vi "test_0.1.0a1.vi"() -> ()   [LabVIEW 2011]
panel:
  in  "meta":string[](array[string])
  in  "Pages":i32
  out "return type 5":i32
  out "return type 4":i32
  out "return type 3":i32
  out "return type 2":i32
  out "return type":i32
  in  "path in":path=path "\\\\vmware-host\\Shared Folders/shared/camtiff/bin/libctiff.dll"
  out "error out":errorcluster
  in  "name":string="LabVIEW"
  in  "image_desc":string="LabVIEW Testing"
  in  "software":string="Make"
  in  "model":string="Model"
  in  "make":string="Make"
  in  "copyright":string="Copyright"
  in  "artist":string="Artist"
  in  "output_file":path=path "\\\\vmware-host\\Shared Folders/shared/camtiff/labview_test.tiff"
  in  "Array":u16[][](array[numeric])=[[0, 0, 0, 0], [0, 24000, 0, 0], [0, 0, 37000, 0], [0, 0, 0, 65535]]
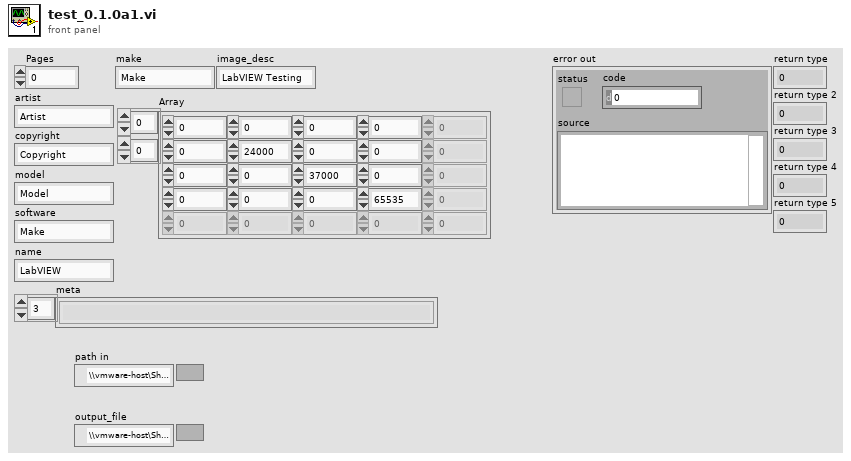
[diagram p1: front panel]
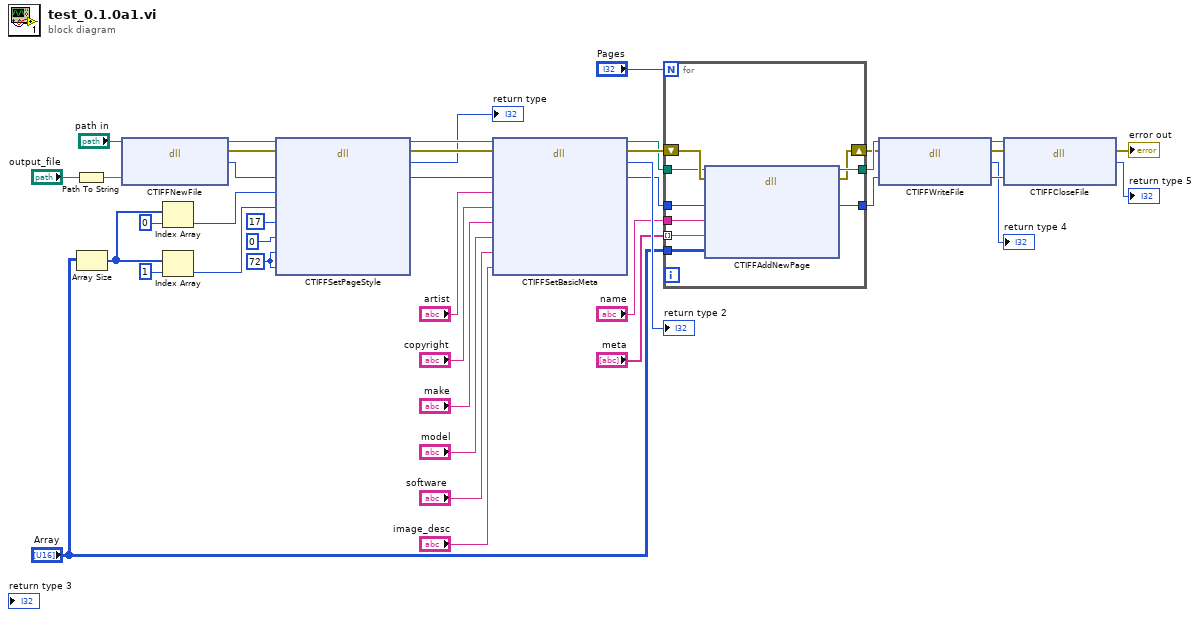
[diagram p0: block diagram]
diagram:
  w25 = u32 72 ("x_resolution")
  n1 = Path To String(path="output_file") -> (string=w15:string)
  n2 = Array Size(array="Array") -> (size(s)=w31:i32[])
  n3 = dll-call lib="\\\\vmware-host\\Shared Folders/shared/camtiff/bin/libctiff.dll" fn="CTIFFNewFile"(path in="path in", "output_file"=w15) -> (path out=w17:path, error out=w23:errorcluster, "return type"=w33:i64)  [unwired: 3 in]
  n4 = Index Array(array=w31, index=0) -> (element=w29:i32)
  n5 = Index Array(array=w31, index=1) -> (element=w28:i32)
  n6 = dll-call lib="?" fn="CTIFFSetPageStyle"(path in=w17, error in=w23, "ctiff"=w33, "width"=w29, "height"=w28, "pixel_type"=u32 17, "in_color"=u8 0, "x_resolution"=w25, "y_resolution"=w25) -> (path out=w35:path, error out=w24:errorcluster, "return type"=→"return type":i32, "ctiff"=w34:i64)  [unwired: 7 in]
  n7 = dll-call lib="?" fn="CTIFFSetBasicMeta"(path in=w35, error in=w24, "ctiff"=w34, "artist"="artist", "copyright"="copyright", "make"="make", "model"="model", "software"="software", "image_desc"="image_desc") -> (path out=w1:path, error out=w3:errorcluster, "return type"=→"return type 2":i32, "ctiff"=w5:i64)  [unwired: 7 in]
  n8 = for {
    N: "Pages" -> [_]
    tunnel: [w50] -> w10
    tunnel: [w49] -> w9
    tunnel: "name" -> [w48]
    tunnel: "Array" -> [w47]
    tunnel: w5 -> [w46]
    tunnel: "meta" -> [w45] mode=indexing
    shift-right: [w43] -> w2
    shift-left: w3 -> [w44]
    tunnel: w1 -> [w42]
    n9 = dll-call lib="?" fn="CTIFFAddNewPage"(path in=w42, error in=w44, "ctiff"=w46, "name"=w48, "meta"=w45, "buffer"=w47) -> (path out=w50:path, error out=w43:errorcluster, "ctiff"=w49:i64)  [unwired: 5 in]
  }
  n10 = dll-call lib="?" fn="CTIFFWriteFile"(path in=w10, error in=w2, "ctiff"=w9) -> (path out=w22:path, error out=w21:errorcluster, "return type"=→"return type 4":i32, "ctiff"=w20:i64)  [unwired: 1 in]
  n11 = dll-call lib="?" fn="CTIFFCloseFile"(path in=w22, error in=w21, "ctiff"=w20) -> (error out=→"error out":errorcluster, "return type"=→"return type 5":i32)  [unwired: 2 in, 1 out]
